vi "Initialize Device Folder.vi"(8 "error in (no error)":errorcluster, 10 "Default Path in":path, 11 "Control Experiment":refnum<class "Control Experiment.lvclass">) -> (0 "error out":errorcluster, 2 "Device Path":path, 3 "Control Experiment out":refnum<class "Control Experiment.lvclass">)   [LabVIEW 2019, in "Control Experiment.lvclass"]
uses:
  Control Experiment.lvclass
  <userlib>/_MGI/File/MGI Create Directory Chain Behavior Enum.ctl
  Control Experiment.lvclass/Control Experiment.ctl
panel:
  in  "Control Experiment":refnum<class "Control Experiment.lvclass">
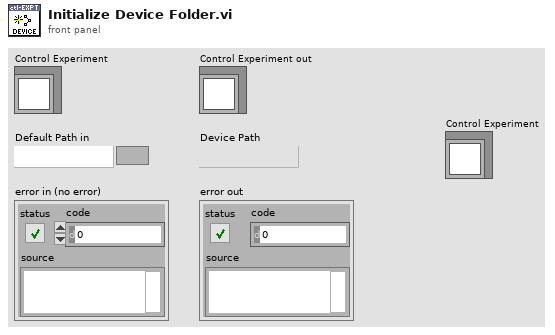
[diagram p1: front panel]
types:
  T1 = typedef "MGI Create Directory Chain Behavior Enum.ctl" = enum16{"Auto Detect", "Path Contains a File", "Path Does Not Contain a File"}
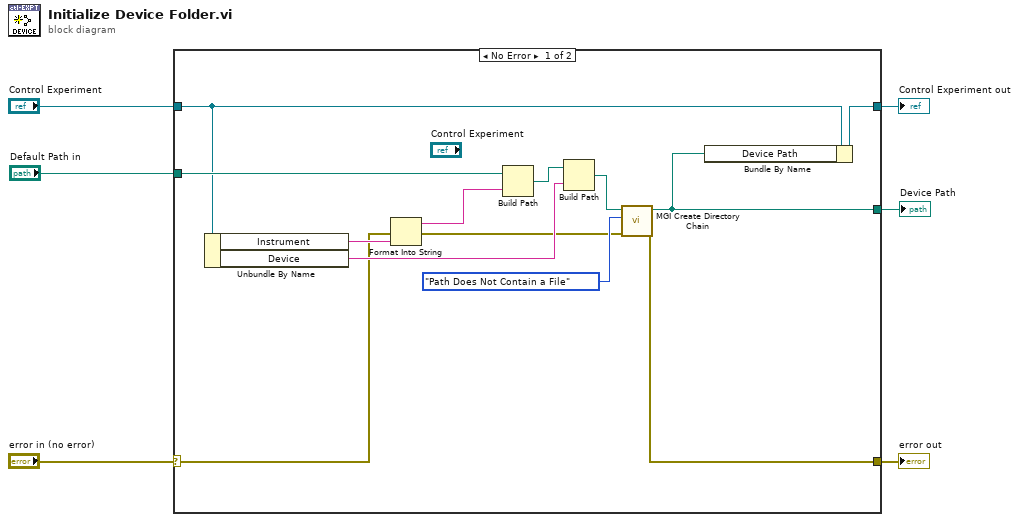
[diagram p0: block diagram]
diagram:
  n1 = case shown="No Error" "error in (no error)" {
    selector: "error in (no error)" -> [w10 w21]
    tunnel: "Control Experiment" -> [w9 w20]
    tunnel: "Default Path in" -> [w13 _]
    tunnel: [w7 _] -> w5
    tunnel: [w11 w21] -> w4
    tunnel: [w8 w20] -> w1
    frame No Error {
      n2 = Unbundle By Name(w9) -> ("Instrument"=w14:string, "Device"=w15:string)
      n3 = Format Into String(error in=w10, w14) -> (resulting string=w18:string, error out=w12:errorcluster)  [unwired: 2 in]
      n4 = Build Path(base path=w13, name or relative path=w18) -> (appended path=w19:path)
      n5 = Build Path(base path=w19, name or relative path=w15) -> (appended path=w17:path)
      n6 = call <userlib>:"MGI Create Directory Chain.vi"("Error In"=w12, "File Presence (Auto Detect)"=MGI_Create_Directory_Chain_Behavior_Enum."Path Does Not Contain a File", "Path"=w17) -> ("Error Out"=w11:errorcluster, "Duplicate Path"=w7:path)  [unwired: 7 in]
      n7 = Bundle By Name(cluster=w9, "Device Path"=w7) -> (w8:refnum<class "Control Experiment.lvclass">)
    }
    frame Error {
    }
  }
  "Device Path" <- w5
  "error out" <- w4
  "Control Experiment out" <- w1
